vi "Read element.vi"(8 "error in":errorcluster, 11 "EIP Tags Channel in":refnum<class "EIP Tags Channel.lvclass">) -> (0 "error out":errorcluster, 2 "element":i32, 3 "EIP Tags Channel out":refnum<class "EIP Tags Channel.lvclass">)   [LabVIEW 2013, in "EIP Tags Channel.lvclass"]
uses:
  EIP Tags Channel.lvclass
  EIP Tags Channel.lvclass/EIP Tags Channel.ctl
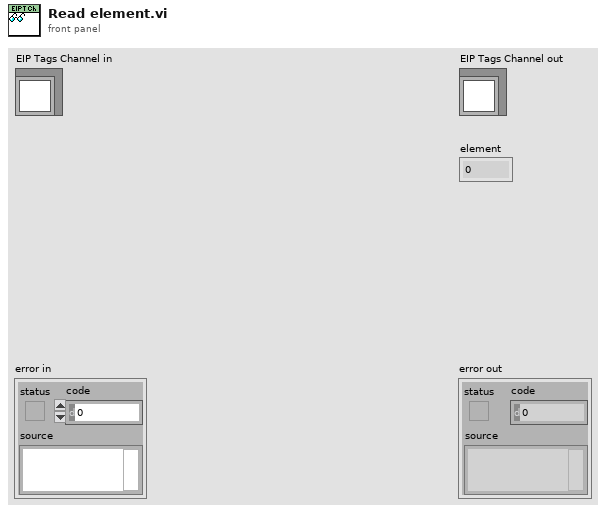
[diagram p1: front panel]
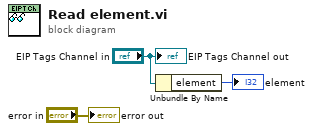
[diagram p0: block diagram]
diagram:
  n1 = Unbundle By Name("EIP Tags Channel in") -> ("element"=→"element":i32)
  "error out" <- "error in"
  "EIP Tags Channel out" <- "EIP Tags Channel in"
